vi "VG CAN VEH ON.vi"() -> ()   [LabVIEW 2020]
panel:
  out "CAN VEH ON":bool
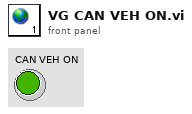
[diagram p1: front panel]
diagram:
